vi "Close.vi"(8 "error in":errorcluster, 11 "Output Enable in":refnum<class "Output Enable.lvclass">) -> (0 "error out":errorcluster, 3 "Output Enable out":refnum<class "Output Enable.lvclass">)   [LabVIEW 2023, in "Output Enable.lvclass"]
uses:
  Output Enable.lvclass
  Capabilities.lvclass
  Output Enable.lvclass/Output Enable.ctl
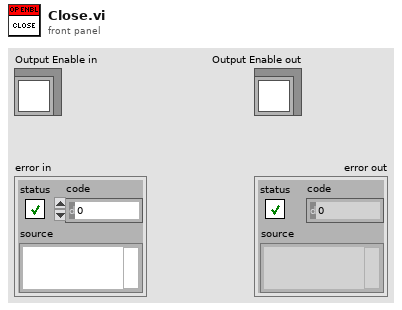
[diagram p1: front panel]
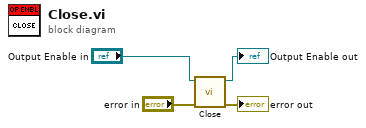
[diagram p0: block diagram]
diagram:
  n1 = call-parent "Close.vi"("error in"="error in", "Capabilities in"="Output Enable in") -> ("error out"=→"error out":errorcluster, "Capabilities out"=→"Output Enable out":refnum<class "Output Enable.lvclass">)  [unwired: 8 in]
